vi "Less Than.vi"(1 "comparable b":refnum<class "Less Comparable.lvclass">, 2 "comparable a":refnum<class "Less Comparable.lvclass">, 3 "Less Functor":refnum<class "Less Functor.lvclass">) -> (0 "less?":bool)   [LabVIEW 2020, in "Less Functor.lvclass"]
doc: "Returns whether <b>comparable a</b> is less than <b>comparable b</b>."
uses:
  <vilib>/Comparison/Less/Less Functor/Less Functor.lvclass
  <vilib>/Comparison/Less/Less Comparable/Less Comparable.lvclass
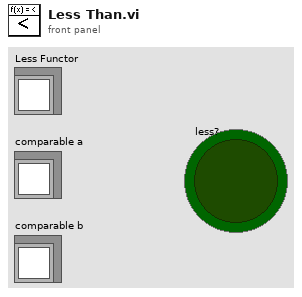
[diagram p1: front panel]
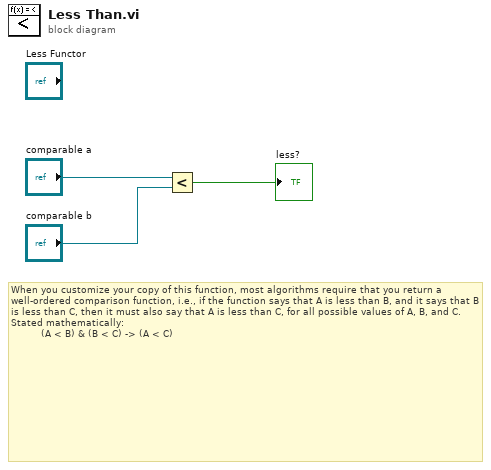
[diagram p0: block diagram]
diagram:
  # "When you customize your copy of this function, most algorithms require that you return a well-ordered comparison function, i.e., if the function says that A is less than B, and it says that B is less than C, then it must also say that A is less than C, for all possible values of A, B, and C. Stated mathematically:\n          (A < B) & (B < C) -> (A < C)"
  n1 = Less?(x="comparable a", y="comparable b") -> (x < y?=→"less?":bool)
